vi "get_objects.vi"(8 "error in (no error)":errorcluster, 11 "HGF_FGV_Delete":refnum<class "HGF_FGV_Delete.lvclass">) -> (0 "error out":errorcluster, 2 "objects":refnum<class>[](array[class]), 3 "dup HGF_FGV_Delete":refnum<class "HGF_FGV_Delete.lvclass">)   [LabVIEW 2012, in "HGF_FGV.lvlib" / "HGF_FGV_Delete.lvclass"]
doc: "Returns the deleted objects."
uses:
  HGF_FGV_Delete.lvclass
  HGF_FGV_Delete.lvclass/HGF_FGV_Delete.ctl
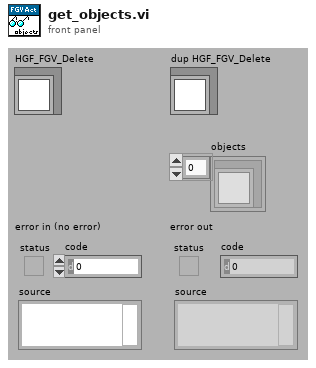
[diagram p1: front panel]
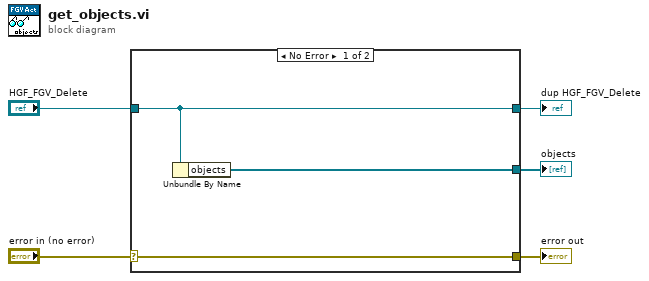
[diagram p0: block diagram]
diagram:
  n1 = case shown="No Error" "error in (no error)" {
    selector: "error in (no error)" -> [w8 w9]
    tunnel: [w8 w9] -> w4
    tunnel: [w7 w10] -> w2
    tunnel: "HGF_FGV_Delete" -> [w7 w10]
    tunnel: [w6 _] -> w1
    frame No Error {
      n2 = Unbundle By Name(w7) -> ("objects"=w6:refnum<class>[])
    }
    frame Error {
    }
  }
  "error out" <- w4
  "dup HGF_FGV_Delete" <- w2
  "objects" <- w1
